vi "unpack_rm_imu.vi"(10 "payload_size":u32, 11 "payload":u64) -> (2 "error":bool, 3 "samples":T1(array[cluster]))   [LabVIEW 2023]
panel:
  in  "rm_imu_sample":T2
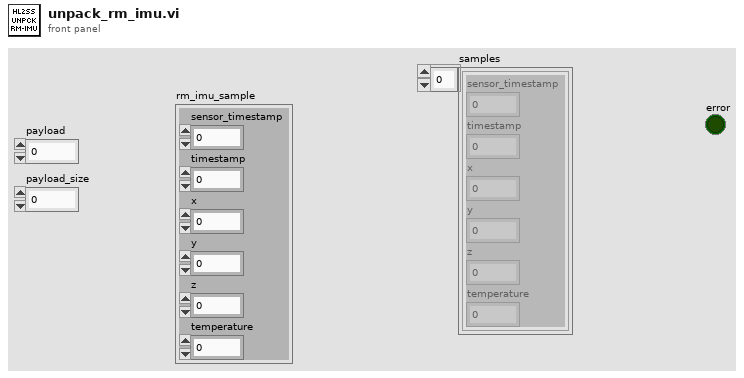
[diagram p1: front panel]
types:
  T1 = cluster{"sensor_timestamp":u64, "timestamp":u64, "x":sgl, "y":sgl, "z":sgl, "temperature":sgl}[]
  T2 = cluster{"sensor_timestamp":u64, "timestamp":u64, "x":sgl, "y":sgl, "z":sgl, "temperature":sgl}
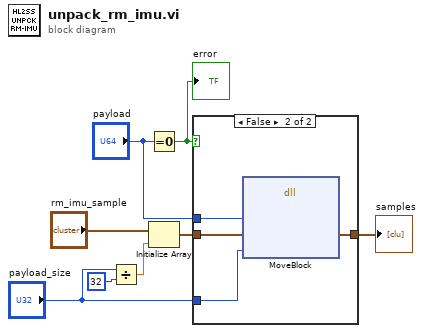
[diagram p0: block diagram]
diagram:
  n1 = Divide(x="payload_size", y=u32 32) -> (x/y=w4:dbl)
  n2 = Equal To 0?(x="payload") -> (x = 0?=w7:bool)
  "error" <- w7
  n3 = Initialize Array("rm_imu_sample", w4) -> (w3:T1)
  n4 = case shown="False" w7 {
    tunnel: "payload" -> [_ w12]
    tunnel: "payload_size" -> [_ w13]
    tunnel: w3 -> [w9 w11]
    tunnel: [w9 w10] -> w1
    frame True {
    }
    frame False {
      n5 = dll-call lib="LabVIEW" fn="MoveBlock"("ps"=w12, "pd"=w11, "size"=w13) -> ("pd"=w10:T1)  [unwired: 6 in, 2 out]
    }
  }
  "samples" <- w1
